vi "scripting_create_vi.vi"(8 "error in (no error)":errorcluster, 10 "Template VI Path":path, 11 "New VI File Path":path) -> (0 "error out":errorcluster)   [LabVIEW 2023]
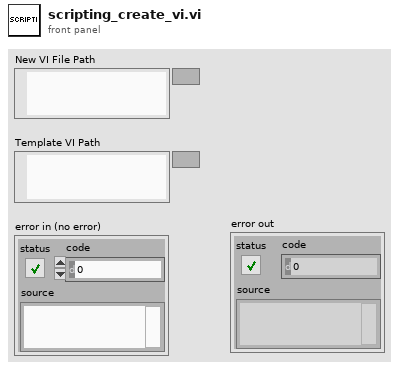
[diagram p1: front panel]
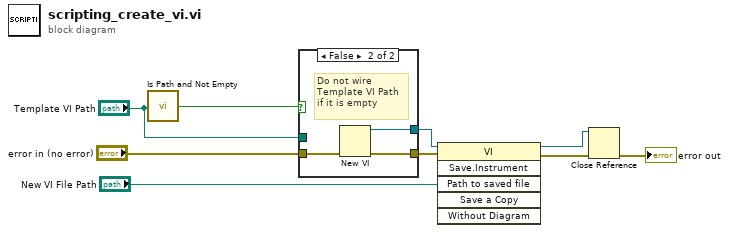
[diagram p0: block diagram]
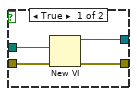
[diagram p2: hidden frame]
diagram:
  n1 = call <vilib>:"Is Path and Not Empty.vi"("path"="Template VI Path") -> ("Is Path and Not Empty?"=w2:bool)  [unwired: 4 in]
  n2 = case shown="False" w2 {
    tunnel: [w13 w16] -> w9
    tunnel: [w12 w15] -> w8
    tunnel: "error in (no error)" -> [w11 w14]
    tunnel: "Template VI Path" -> [w10 _]
    frame True {
      n3 = New VI(8:w11, 10:w10) -> (0:w13:errorcluster, 3:w12:refnum<vi>)  [unwired: 5 in]
    }
    frame False {
      # "Do not wire\nTemplate VI Path\nif it is empty"
      n4 = New VI(8:w14) -> (0:w16:errorcluster, 3:w15:refnum<vi>)  [unwired: 6 in]
    }
  }
  n5 = invoke class="VI" method="Save.Instrument"(reference=w8, error in=w9, "Path to saved file"="New VI File Path") -> (reference out=w3:refnum<vi>, error out=w5:errorcluster)  [unwired: 3 in, 4 out]
  n6 = Close Reference(reference=w3, error in (no error)=w5) -> (error out=→"error out":errorcluster)
